vi "Main_23b.vi"() -> ()   [LabVIEW 2020]
uses:
  RB ENUM_Spot ID.ctl
  Cluster _Point Location.ctl
  ENUM_Location Direction.ctl
panel:
  out "rounds":i32
  out "Elf Locations":T1[](array[typedef])
  out "Grove":T2[][](array[typedef])
  in  "Example 2":string="....#..\n..###.#\n#...#.#\n.#...##\n#.###..\n##.#.##\n.#..#.."
  in  "Puzzle":string="###.###...#.##.###.##.###.....#...##.#####..####..#####.#...###..##...#..\n####.#..#..#..#.###..###....###.....#.#.##.###.#..#..#..##########..#..#.\n.##..##..#.##.#.....##.##..#..###..#..#.####...##...#...##.#...#.#....###\n###.#..#.#..#...###.#...#..##.#.#####..#...###.##..#....##..#......##..#.\n.#..##.#.##..##.####.###.###...###.##.#.###.#...####.#######..#..##.#####\n#...#.#.#####...#.#...###...#.#....#..#..##....##...####.####..#.########\n#..######..#.#..#..##......#..##.######....#.....###..######...#.#.###...\n.###.####.#.#.###.#.....#...##..#...#.#.#.#.####.#..#..#.##..##..##.#.#.#\n#.#..#.####....#.##.#........#....#.###.##...##......#...#..####.#.#.#.#.\n###.#..##...#.#.#.##.##....#.#..#....######...#...##.#.####..#...##.#..#.\n#...###..#.##..#.#.#...##..#.#.....#..#..#.#...#...#####..#.##..#.##.####\n..#.#.#....#..#..###.#...#.#..#.#.#..#....###...###......#.#.#...#.######\n###.###.###.#.#...####.###..#.#..#....#..#.###........#....##.#.....###..\n#..#..#..#.###...#.##.##...#.##.#.#.#.#.###.#.##..#..##.#.####.#####..#.#\n.###.##..###.....#.#..#.#..###..#.#..#.#...##.#.....##...####..#.#.##.##.\n#.###.##.##.####.###.#.#.#..##..####...#####...###..#.##..##.##.###.##.#.\n#.####.####.#..#######..###...#.....##.###.#.##.#.##.###.....#..#..#...#.\n..###.##..######..#....#.#.#....#..#..#.#.####..#....####.##.##.#.#######\n#..##.#..####..######.####.#..#.#..##...###.###.####.#.....##.#####..##..\n.##..#...##..###..####.##.########.#.#....#.##..##.#.........#...########\n##..###..#....#.###.##.#.#...###.###.##.#...##..#..#.###.##.#.##...##...#\n.#...##.###..#.########.#....#.##......#...#.##..##..#.###..##.......##.#\n#.#.....#####..#.#..#####.##..###..#.##.##..#..#.......##.#.##.##..######\n#.##.#.##.###.#..########..##.#.#.#######....###.....###.#...#.##....##..\n.#..#...#.###.#.#..#..#.....#..##...##.#.#####.#...##....##...#.......###\n...#...#####..########.####.######.####..#.#.#.##.#.###...#.##.###..#...#\n.#.#.####.###...##.####.......#..#..#...#......######.##.#...#.#...######\n#.....##.###.###.###.##.....#..#######....#..#.#...##.#..#..###.#..#.#..#\n.#...##.#...###.###.##...##..#.#.####.#.##..#.##.#.#.####....#.#.#.#.####\n.#######.#.....##.####...##..##.###...##.##.#..#..#...#..#####.#.###..##.\n....##.......#...#.###.#####..#.#.##.#.#.##..#.##.#####.##.##.#..##.###..\n###.#.##...#.#.####.####..##...##..##.#.#.#.#...###.##.###.##..#...#...#.\n.#.##.#....##..#.##...##.###..###..#.#..#.#########.....#.##...##....#.#.\n..##.#..###..#.......#....#.#.#.###.###.#.#..#.#.#..#...#.###.##..####...\n.##.##.#.###...#.##....#.##..###..#..###..###.#...##.....#.###.#.####..#.\n....#..##..#.......####.##.#.##.###.#.#..######.###.##.#.#.###..####..#..\n####..#.###.##..##.##..#.###....####.###.#.#####.#.##.#.#...##.....##...#\n.#....#.##...#....#####....#.#######.#.###...###.#.##.#..#.##...#.#....#.\n#.###..####......###.##....#.#.####...#.#.#...###.#.........#.#.##......#\n#..#....#.#.##..##..#..#.###.###.#.###.#####..#..##.###...##.##..#.#....#\n#...##.#...##.#.##...##.#..#.#.##.##....#....#..##..###.#....####.######.\n....#.#...##.......#####...######..###...###.##.#.##.#.##..#.##.##....#..\n..####.###..#....##.##.############.#.##...####.###.#....#....##.#.######\n#...#.#####.#.##.#.##.##...###.....#..###.#.###.###........#....#...#....\n#...#....#...####..#.#..###....#..#######.#....##..##..#..#..##..#...####\n#.#.##.##.##.#.##.####..####.....##.....#.#.#.##..###.#.##.#...##.#..##..\n..#..##.#..###.....##.##...#.##..#.##...###.#.###.#..###.....#..##..#..##\n##.#.#.#.###...#....##.....######..#####.##..#..#..#.##.#.####..##.##.##.\n.##.##...#.##.#...##...####.#..#...#.#..#.###.##.##....#.##.#..#..#.#.###\n.###.#...###.##.#.#..###.##..###.#####.#..#####..###....###.##.#.#.#..###\n..###...#####...#...##..#.#.#...#.##....#..##.#..#.#.#...####..#.#.##..#.\n#.#.##.##.#.##...##.#.##.##.#.##.###..###..#.##..#.#..####.##.#.....##..#\n..#..###..#.#####..###.##......####.###..#.##.#.##..###..#.###..#####.#..\n.###.#...#.#.#.#####..###..###.#..##.###..##...###.#.#..#....##.#.#.##.#.\n#.##....####.##.##...###.##...######....#..##.#.#..#####...#...#.###.##..\n..#....##...#.#####....#......#.....#.#.#...#...#...##.#.#...##..#.#...##\n.#.#..##..######..##..#.#..#.........#.#..#....#.#......#.##..###.##.#..#\n####..#.#.#..#..##..#.#.####.###......#..#.....#..#.####..#.#####.#..#.##\n.##.#..##..###....#..#...#.#####....##..#......###...##.#...##....####..#\n..####.#..###.###.###...##..#.#......#####.#.#.#..##......###.#.#.###.##.\n#####....###.##..#.##..###########..#.#.#.#...##..#####.#.#..#..####..#.#\n##..#.##.#.##.....#.###.#.#.......##...#...#.#.##....#..#......#####..##.\n###.#...##.##..####.#...####..#.###.....#.###...#.#.##..#####......#.#.##\n#.##.#############.##....#.###.####.##.#.######.#.#....#..######..##.####\n.#.###.####.##...#..##....##..##.#..#.#...#####...####....#..#...###.#.#.\n.###..#..##...##..####...###.#..##########.###.##.#..###.#..###...##.#.##\n.##.##.#..#.####..#####......##.#..#....#.##..#.####.#.###########.#.#.#.\n..#.####.#...##.#.#....##.#...##..##...#.#.#.##..##..##.####..##.#####.#.\n.....#.##.####..##.#.##....#.##..##..##...#.#...##..#.#..####.###..#.#..#\n..#.....#####.##..###.#.###.....#.#.######.#.....###.....#..#.#...#..#.##\n#.#..#.#..##.#.#.....##.#.##..###.###.##..#..###..######..#.####.....##.#\n..####.......###.#..###.#.#.######.####.##...#.##...######..#####...#...#\n#.#.####.####..########.#.....##......#.##.##.#.#....##.####.##..#...####"
  in  "Example":string=".....\n..##.\n..#..\n.....\n..##.\n....."
  # "--- Part Two ---\nIt seems you're on the right track. Finish simulating the process and figure out where the Elves need to go. How many rounds did you save them?\n\nIn the example above, the first round where no Elf moved was round 20:\n\n.......#......\n....#......#..\n..#.....#.....\n......#.......\n...#....#.#..#\n#.............\n....#.....#...\n..#.....#.....\n....#.#....#..\n.........#....\n....#......#..\n.......#......\nFigure out where the Elves need to go. What is the number of the first round where no Elf moves?"
  # "1057"
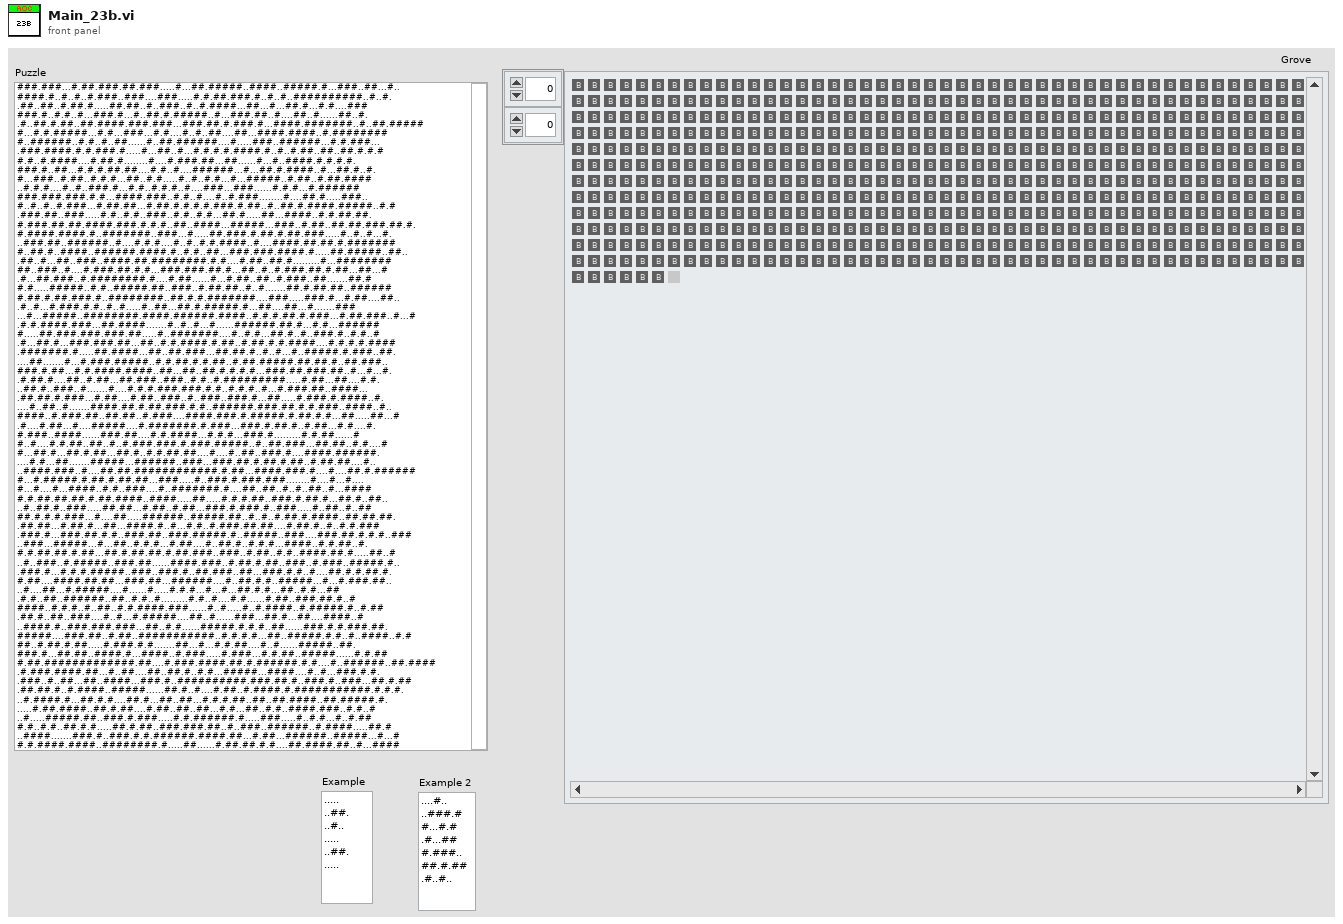
[diagram p1: front panel]
types:
  T1 = typedef "Cluster _Point Location.ctl" = cluster{"X col":i32, "Y row":i32}
  T2 = typedef "RB ENUM_Spot ID.ctl" = enum32{"Blank", "ELF", "Proposed"}
  T3 = typedef "ENUM_Location Direction.ctl" = enum16{"North", "North-East", "East", "South-East", "South", "South-West", "West", "North-West", "Center"}
  T4 = typedef "MAP_Poroposed Moves.ctl" = map{T1, cluster{"Elf":i32, "move":bool}}
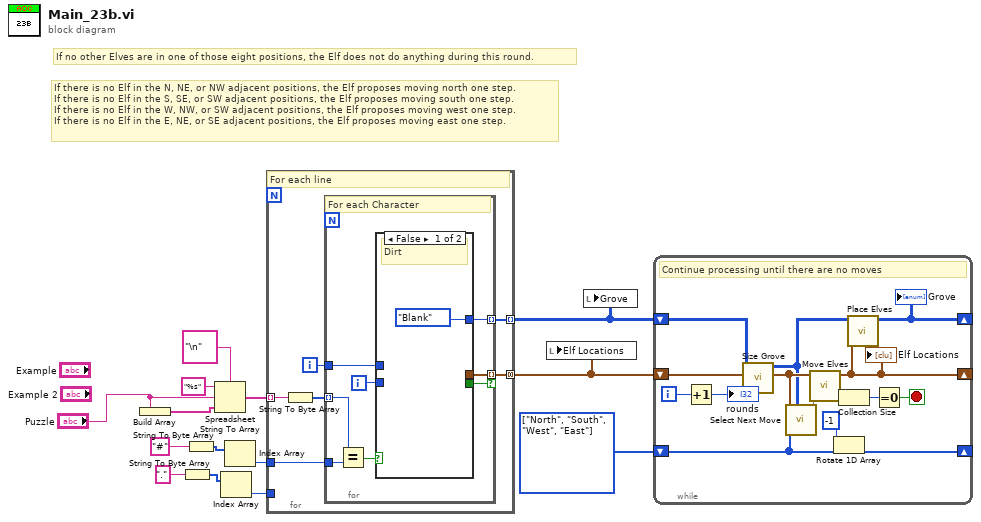
[diagram p0: block diagram]
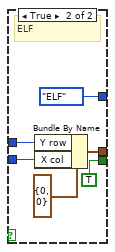
[diagram p2: hidden frame]
diagram:
  w4 = T3[] [enum."North", enum."South", enum."West", enum."East"] items=["North", "North-East", "East", "South-East", "South", "South-West", "West", "North-West", "Center"] ("Array")
  # "If there is no Elf in the N, NE, or NW adjacent positions, the Elf proposes moving north one step.\nIf there is no Elf in the S, SE, or SW adjacent positions, the Elf proposes moving south one step.\nIf there is no Elf in the W, NW, or SW adjacent positions, the Elf proposes moving west one step.\nIf there is no Elf in the E, NE, or SE adjacent positions, the Elf proposes moving east one step."
  # "If no other Elves are in one of those eight positions, the Elf does not do anything during this round."
  n1 = Build Array("Puzzle") -> (w14:string[])
  n2 = String To Byte Array(string="." ("format string")) -> (unsigned byte array=w7:u8[])
  n3 = String To Byte Array(string="#" ("format string")) -> (unsigned byte array=w8:u8[])
  n4 = Spreadsheet String To Array(delimiter (Tab)="\n", format string="%s", spreadsheet string="Puzzle", array type (2D Dbl)=w14) -> (array=w11:string[])
  n5 = Index Array(array=w7) -> (element=w6:u8)  [unwired: 1 in]
  n6 = Index Array(array=w8) -> (element=w5:u8)  [unwired: 1 in]
  n7 = for {
    tunnel: w11 -> [w20] mode=indexing
    tunnel: w6 -> [_]
    tunnel: w5 -> [w18]
    tunnel: [w17] -> w3 mode=indexing
    tunnel: [w15] -> w2 mode=concatenating
    i -> [w16]
    # "For each line"
    n8 = String To Byte Array(string=w20) -> (unsigned byte array=w19:u8[])
    n9 = for {
      tunnel: w19 -> [w27] mode=indexing
      tunnel: w18 -> [w28]
      tunnel: [w25] -> w17 mode=indexing
      tunnel: w16 -> [w23]
      tunnel: [w22] -> w15 mode=indexing if=w21
      i -> [w24]
      # "For each Character"
      n10 = Equal?(x=w27, y=w28) -> (x = y?=w26:bool)
      n11 = case shown="False" w26 {
        tunnel: [RB_ENUM_Spot_ID."Blank" ("Spot") RB_ENUM_Spot_ID."ELF" ("Spot")] -> w25
        tunnel: w24 -> [_ w33]
        tunnel: w23 -> [_ w32]
        tunnel: [_ w31] -> w22
        tunnel: [_ TRUE] -> w21
        frame False {
          # "Dirt"
        }
        frame True {
          # "ELF"
          n12 = Bundle By Name(cluster=T1 {"X col"=0, "Y row"=0} ("Point"), "Y row"=w32, "X col"=w33) -> (w31:T1)
        }
      }
    }
  }
  n13 = local write "Elf Locations"(w2) -> ()
  n14 = local write "Grove"(w3) -> ()
  n15 = while {
    shift-right: [w45] -> _
    shift-left: w3 -> [w46]
    shift-right: [w44] -> _
    shift-left: w2 -> [w43]
    shift-right: [w49] -> _
    shift-left: w4 -> [w47]
    i -> [w40]
    stop <- w36 stop-if-true
    # "Continue processing until there are no moves"
    n16 = Increment(x=w40) -> (x+1=→"rounds":i32)
    n17 = call "Size Grove.vi"("Elf Locations"=w43, "Original Grove"=w46) -> ("Elf Locations 2"=w42:T1[], "Spaced Grove"=w41:T2[][])  [unwired: 8 in]
    n18 = call "Select Next Move.vi"("Grove"=w41, "Proposed Direction List"=w47, "Elf"=w42) -> ("propose Moves"=w38:T4)  [unwired: 7 in, 1 out]
    n19 = call "Move Elves.vi"("propose Moves"=w38, "Elf Positions"=w42) -> ("New Elf Positions"=w44:T1[])  [unwired: 9 in]
    "Elf Locations" <- w44
    n20 = Rotate 1D Array(1:w47, 2:-1 ("n")) -> (0:w49:T3[])
    n21 = Collection Size(1:w38) -> (0:w37:i32)
    n22 = call "Place Elves.vi"("Elf Locations"=w44, "Spaced Grove in"=w41) -> ("Spaced Grove out"=w45:T2[][])  [unwired: 9 in]
    "Grove" <- w45
    n23 = Equal To 0?(x=w37) -> (x = 0?=w36:bool)
  }
